vi "Circle.vi"(4 "Properties":T1={"Color"=2147483647, "Line"={"Style"=enum."Automatic", "Color"=2147483647, "Width"=nan}, "Display"={"Alpha"=nan, "Z Order"=nan}} {"Color" items=["Automatic"=2147483647, "Black"=0, "White"=16777215, "Red"=16711680, "Green"=2263842, "Blue"=255, "Cyan"=65535, "Magenta"=16711935, "Yellow"=16776960]; "Line"."Color" items=["Automatic"=2147483647, "Black"=0, "White"=16777215, "Red"=16711680, "Green"=2263842, "Blue"=255, "Cyan"=65535, "Magenta"=16711935, "Yellow"=16776960]}, 7 "Radius":dbl, 8 "error in (no error)":errorcluster, 9 "Y Position":dbl, 10 "X Position":dbl, 11 "Plot ID":T6 format="%x") -> (0 "error out":errorcluster, 3 "Plot ID Out":T6 format="%x")   [LabVIEW 2013, in "Advanced Plotting Toolkit.lvlib"]
doc: "Draw a circle on the figure, in data coordinates."
uses:
  Advanced Plotting Toolkit.lvlib
  typedefs/PlotID.ctl
  ShapeProperties.ctl
  typedefs/PlotColor.ctl
  properties/Line.ctl
  properties/Line_Style.ctl
  properties/Display.ctl
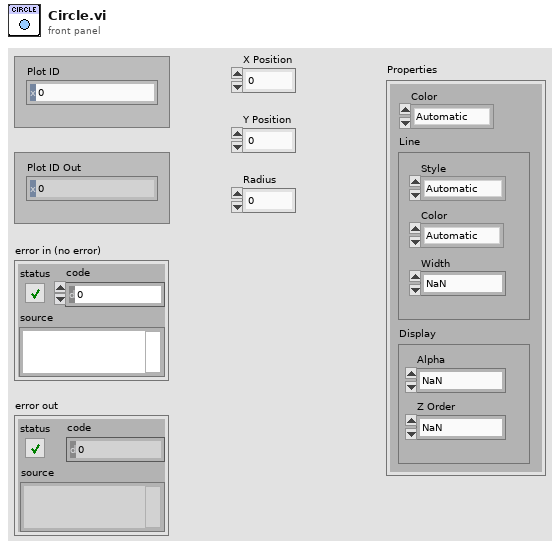
[diagram p1: front panel]
types:
  T1 = typedef "Advanced Plotting Toolkit.lvlib/ShapeProperties.ctl" = cluster{"Color":T2, "Line":T3, "Display":T5}
  T2 = typedef "Advanced Plotting Toolkit.lvlib/PlotColor.ctl" = u32
  T3 = typedef "Advanced Plotting Toolkit.lvlib/Line.ctl" = cluster{"Style":T4, "Color":T2, "Width":sgl}
  T4 = typedef "Advanced Plotting Toolkit.lvlib/Line_Style.ctl" = enum16{"Automatic", "Solid", "Dashed", "Dotted", "Dash-dot", "Invisible"}
  T5 = typedef "Advanced Plotting Toolkit.lvlib/Display.ctl" = cluster{"Alpha":dbl, "Z Order":dbl}
  T6 = typedef "Advanced Plotting Toolkit.lvlib/PlotID.ctl" = i32
  T7 = typedef "Advanced Plotting Toolkit.lvlib/KeyValue.ctl" = cluster{"Key":string, "Value":string}
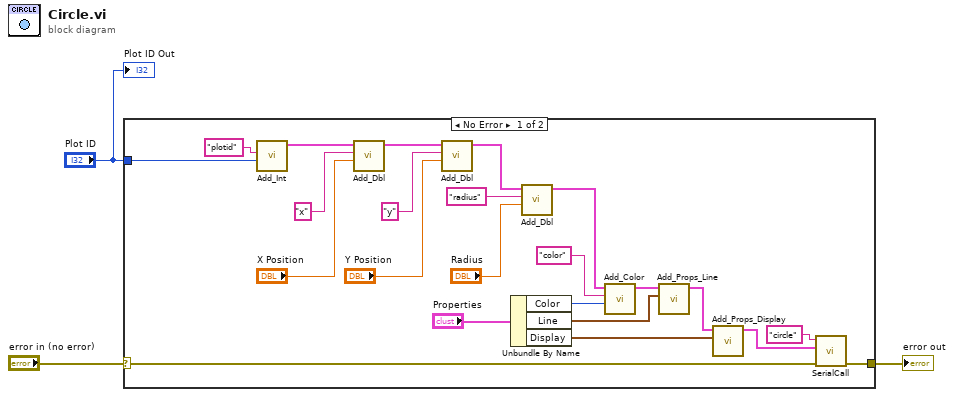
[diagram p0: block diagram]
diagram:
  n1 = case shown="No Error" "error in (no error)" {
    selector: "error in (no error)" -> [w25 w27]
    tunnel: "Plot ID" -> [w26 _]
    tunnel: [w24 w27] -> w1
    frame No Error {
      n2 = call "Add_Int.vi"("Value"=w26, "Key"="plotid") -> ("Keyword Array Out"=w15:T7[])  [unwired: 9 in]
      n3 = call "Add_Dbl.vi"("Value"="X Position", "Key"="x", "Keyword Array"=w15) -> ("Keyword Array Out"=w14:T7[])  [unwired: 8 in]
      n4 = call "Add_Dbl.vi"("Value"="Y Position", "Key"="y", "Keyword Array"=w14) -> ("Keyword Array Out"=w13:T7[])  [unwired: 8 in]
      n5 = Unbundle By Name("Properties") -> ("Color"=w11:T2, "Line"=w9:T3, "Display"=w8:T5)
      n6 = call "Add_Dbl.vi"("Value"="Radius", "Key"="radius", "Keyword Array"=w13) -> ("Keyword Array Out"=w7:T7[])  [unwired: 8 in]
      n7 = call "Add_Color.vi"("Color"=w11, "Key"="color", "Keyword Array"=w7) -> ("Keyword Array Out"=w6:T7[])  [unwired: 8 in]
      n8 = call "Add_Props_Line.vi"("Line"=w9, "Keyword Array"=w6) -> ("Keyword Array Out"=w5:T7[])  [unwired: 9 in]
      n9 = call "Add_Props_Display.vi"("Display"=w8, "Keyword Array"=w5) -> ("Keyword Array Out"=w4:T7[])  [unwired: 9 in]
      n10 = call "SerialCall.vi"("error in (no error)"=w25, "data"=w4, "Resource"="circle") -> ("error out"=w24:errorcluster)  [unwired: 7 in, 1 out]
    }
    frame Error {
    }
  }
  "error out" <- w1
  "Plot ID Out" <- "Plot ID"
